vi "adder (SubVI).vi"(10 "Numeric 2":dbl, 11 "Numeric":dbl) -> (3 "Numeric 3":dbl)   [LabVIEW 2018]
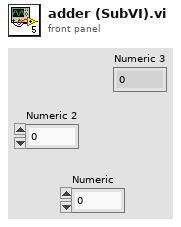
[diagram p1: front panel]
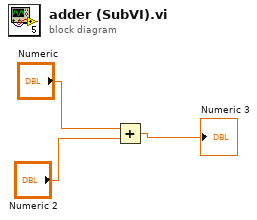
[diagram p0: block diagram]
diagram:
  n1 = Add(x="Numeric", y="Numeric 2") -> (x+y=→"Numeric 3":dbl)
